vi "占空比输出.vi"() -> ()   [LabVIEW 2020]
uses:
  Global_Variable/Global.vi
panel:
  in  "duty cycle":dbl=50.0 format="%#_13g"
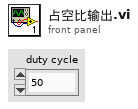
[diagram p1: front panel]
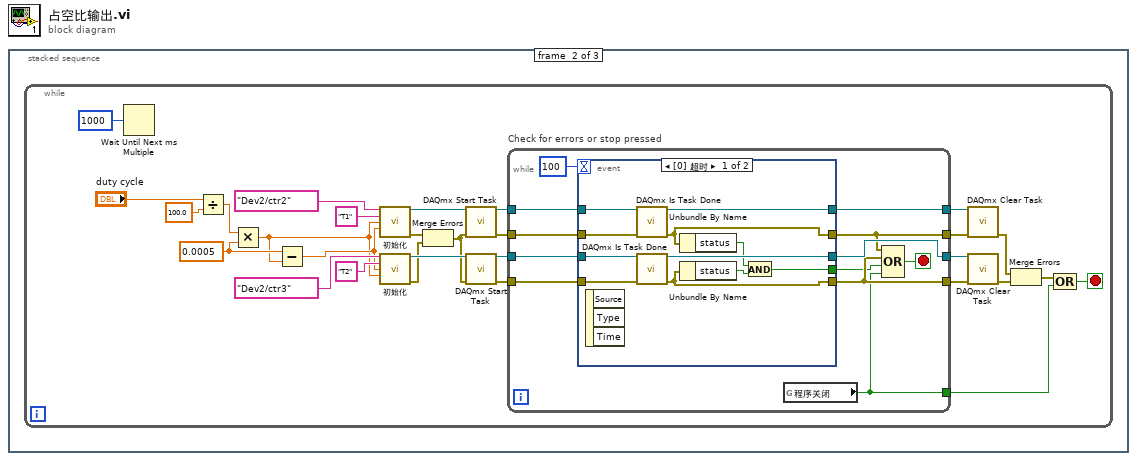
[diagram p0: block diagram]
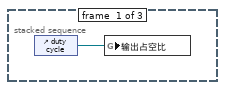
[diagram p2: hidden frame]
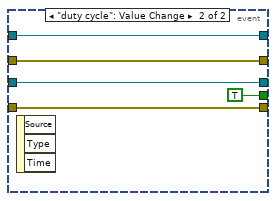
[diagram p3: hidden frame]
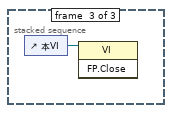
[diagram p4: hidden frame]
diagram:
  n1 = stacked-sequence {
    frame #0 {
      n2 = control-ref of="duty cycle"() -> (w1:refnum<vi>)
      n3 = global write "Global.vi" "输出占空比"(w1) -> ()
    }
    frame #1 {
      n4 = while {
        stop <- w2 stop-if-true
        w19 = 0.0005 ("y")
        n5 = Wait Until Next ms Multiple(millisecond multiple=u32 1000 ("毫秒倍数")) -> ()  [unwired: 1 out]
        n6 = Divide(x="duty cycle", y=100.0) -> (x/y=w20:dbl)
        n7 = Multiply(x=w20, y=w19) -> (x*y=w17:dbl)
        n8 = Subtract(x=w19, y=w17) -> (x-y=w18:dbl)
        n9 = call "初始化.vi"("counter"=tag "Dev2/ctr2", "channel name"="T1", "low time"=w17, "high time"=w18) -> ("task out"=w28:refnum<k21>, "error out"=w9:errorcluster)  [unwired: 10 in]
        n10 = call "初始化.vi"("counter"=tag "Dev2/ctr3", "channel name"="T2", "low time"=w18, "high time"=w17) -> ("task out"=w27:refnum<k21>, "error out"=w8:errorcluster)  [unwired: 10 in]
        n11 = Merge Errors(w9, w8) -> (w7:errorcluster)
        n12 = call <vilib>:"DAQmx Start Task.vi"("task/channels in"=w28, "error in"=w7) -> ("task out"=w30:refnum<k21>, "error out"=w11:errorcluster)  [unwired: 12 in]
        n13 = call <vilib>:"DAQmx Start Task.vi"("task/channels in"=w27, "error in"=w7) -> ("task out"=w15:refnum<k21>, "error out"=w14:errorcluster)  [unwired: 12 in]
        n14 = while "Check for errors or stop pressed" {
          tunnel: [w41] -> w29
          tunnel: w30 -> [w42]
          tunnel: w15 -> [w39]
          tunnel: w14 -> [w38]
          tunnel: [w37] -> w13
          tunnel: [w34] -> w12
          tunnel: w11 -> [w36]
          tunnel: [w35] -> w10
          tunnel: [w31] -> w3
          stop <- w32 stop-if-true
          n15 = event shown="[0] 超时" {
            selector: _ -> [_ _]
            dyn-events: _ -> [_ _]
            timeout: 100 -> [_ _]
            tunnel: w42 -> [w53 w58]
            tunnel: [w52 w58] -> w41
            tunnel: w36 -> [w51 w57]
            tunnel: [w50 w57] -> w35
            tunnel: w39 -> [w49 w54]
            tunnel: w38 -> [w48 w55]
            tunnel: [w47 w54] -> w37
            tunnel: [w46 w55] -> w34
            tunnel: [w43 TRUE ("status")] -> w33
            event Timeout {
              n16 = event-data() -> ()  [unwired: 1 in, 3 out]
              n17 = call <vilib>:"DAQmx Is Task Done.vi"("task/channels in"=w53, "error in"=w51) -> ("task out"=w52:refnum<k21>, "error out"=w50:errorcluster)  [unwired: 11 in, 1 out]
              n18 = call <vilib>:"DAQmx Is Task Done.vi"("task/channels in"=w49, "error in"=w48) -> ("task out"=w47:refnum<k21>, "error out"=w46:errorcluster)  [unwired: 11 in, 1 out]
              n19 = Unbundle By Name(w50) -> ("status"=w45:bool)
              n20 = Unbundle By Name(w46) -> ("status"=w44:bool)
              n21 = And(x=w45, y=w44) -> (x .and. y?=w43:bool)
            }
            event "duty cycle": Value Change {
              n22 = event-data() -> ()  [unwired: 1 in, 3 out]
            }
          }
          n23 = global read "Global.vi" "程序关闭"() -> (w31:bool)
          n24 = Compound Arithmetic op=OR(w35, w34, w33, w31) -> (w32:bool)
        }
        n25 = call <vilib>:"DAQmx Clear Task.vi"("task in"=w29, "error in"=w10) -> ("error out"=w6:errorcluster)  [unwired: 13 in]
        n26 = call <vilib>:"DAQmx Clear Task.vi"("task in"=w13, "error in"=w12) -> ("error out"=w5:errorcluster)  [unwired: 13 in]
        n27 = Merge Errors(w6, w5) -> (w4:errorcluster)
        n28 = Compound Arithmetic op=OR(w4, w3) -> (w2:bool)
      }
    }
    frame #2 {
      n29 = control-ref of="本VI"() -> (w59:refnum<vi>)
      n30 = invoke class="VI" method="FP.Close"(reference=w59) -> ()  [unwired: 2 in, 3 out]
    }
  }
